vi "SRV_Watchdog State Machine.vi"(7 "Cancelled?":bool, 8 "error in (no error)":errorcluster, 10 "TCP Read semaphore":T1, 11 "SRV IP Address":string) -> (0 "error out":errorcluster)   [LabVIEW 2014]
doc: "Author: Mike Schultz (LogicPD, Inc)"
uses:
  Support/SRV_Command-Data Queue Data Type.ctl
  SRV_Watchdog State Machine Local Data.ctl
  SubVIs/SysConfig/SRV_System Config.ctl
  SRV_Watchdog Config Cluster.ctl
  Motors/Motors Config/SRV_Motor Control Command Config.ctl
  <vilib>/Utility/error.llb/DialogType.ctl
panel:
  out "i":i32
  out "Command History":string[](array[string])
  out "Command":string
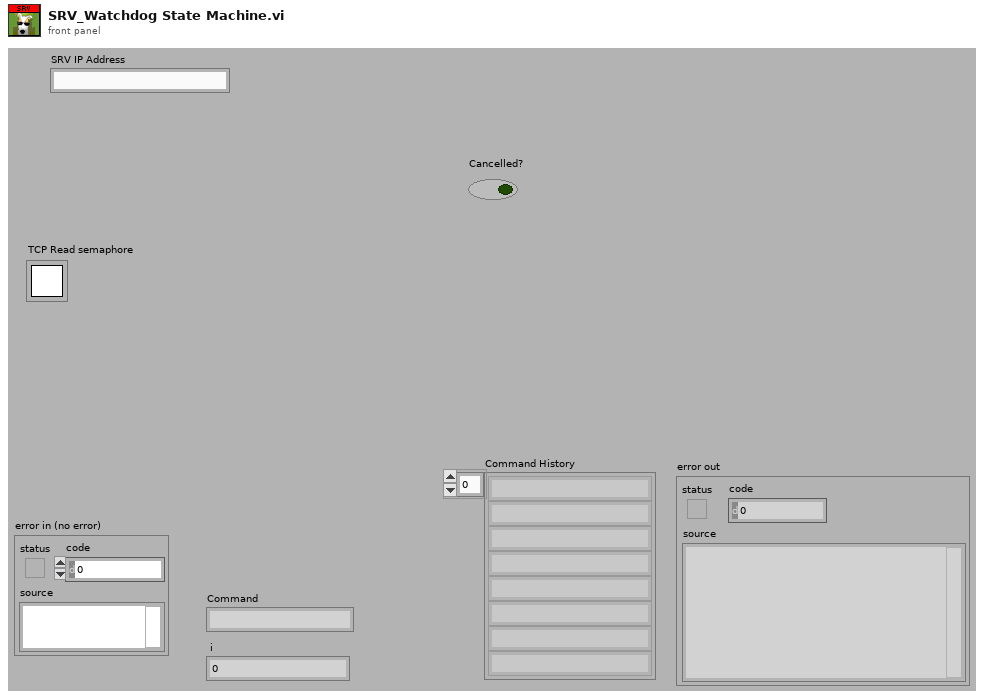
[diagram p1: front panel]
types:
  T1 = typedef "Semaphore RefNum" = refnum<k1>
  T2 = typedef "SRV_Watchdog State Machine Local Data.ctl" = cluster{"SRV IP Address":string, "TCP Read semaphore":T1, "System Config":T3, "WD 1 Last Update":dbl, "WD 2 Last Update":dbl, "SRV":refnum<k5>}
  T3 = typedef "SRV_System Config.ctl" = cluster{"SRV IP Address":string, "Video Stream Rate Period (ms)":u32, "Enable Diagnostic Log":bool, "Watchdog 1 Config":T4, "Watchdog 2 Config":T4, "Sensor Window Filepath":path}
  T4 = typedef "SRV_Watchdog Config Cluster.ctl" = cluster{"Watchdog Name":string, "Watchdog Period (s)":dbl, "Watchdog Command":T5}
  T5 = typedef "SRV_Motor Control Command Config.ctl" = cluster{"I2C Address":u8, "Register":u8, "Value":u8, "Active":bool}
  T6 = typedef "SRV_Command-Data Queue Data Type.ctl" = cluster{"Command":string, "Data":variant}
  T7 = typedef "DialogType.ctl" = u16
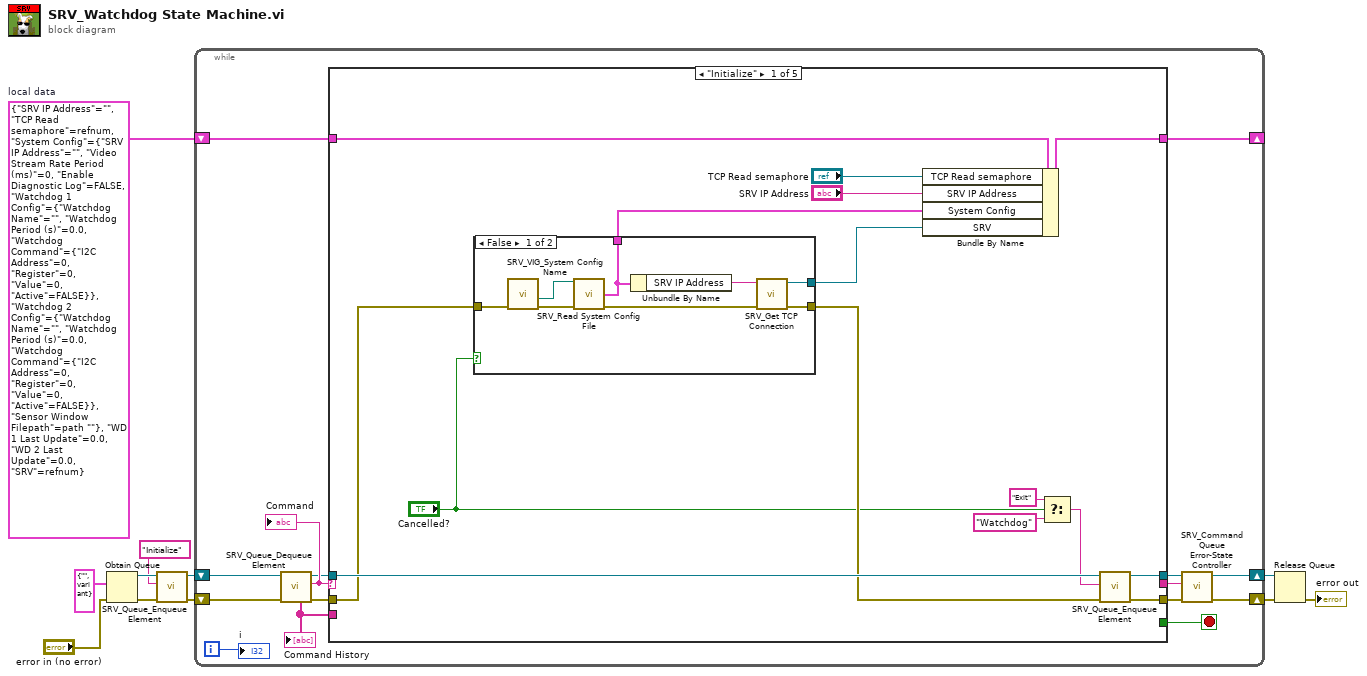
[diagram p0: block diagram]
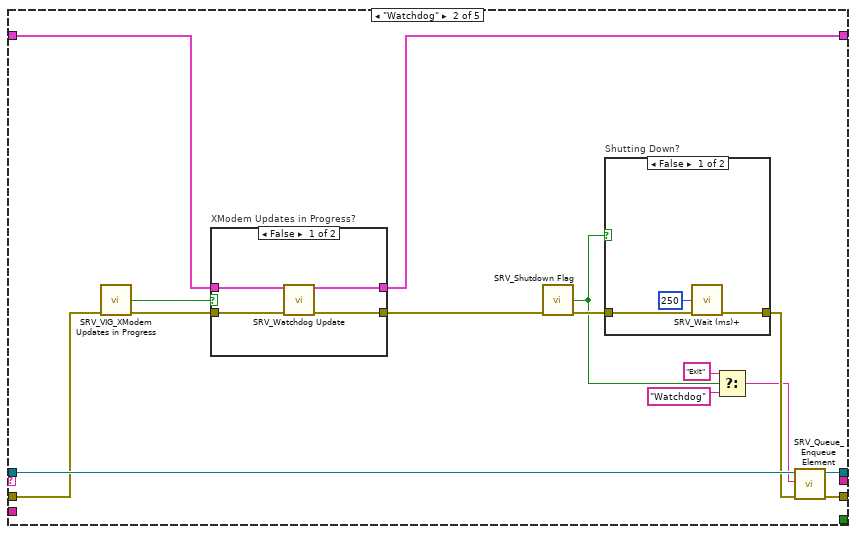
[diagram p3: hidden frame]
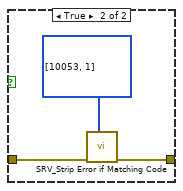
[diagram p5: hidden frame]
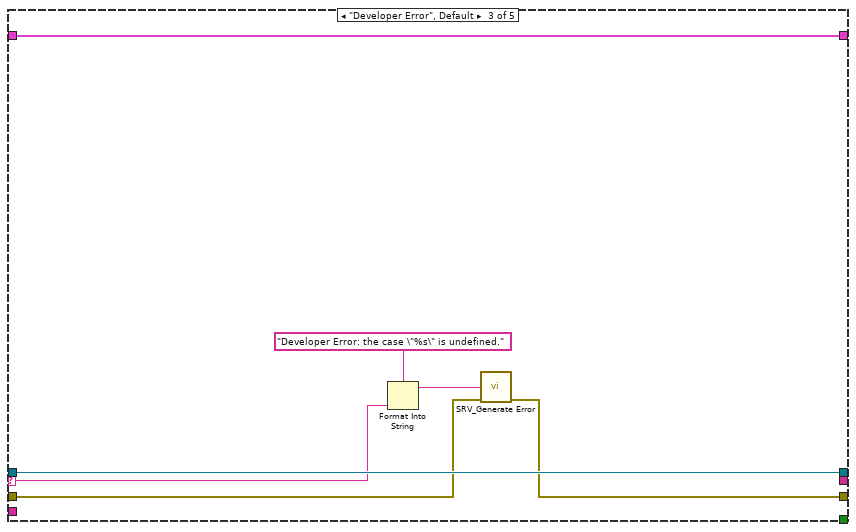
[diagram p6: hidden frame]
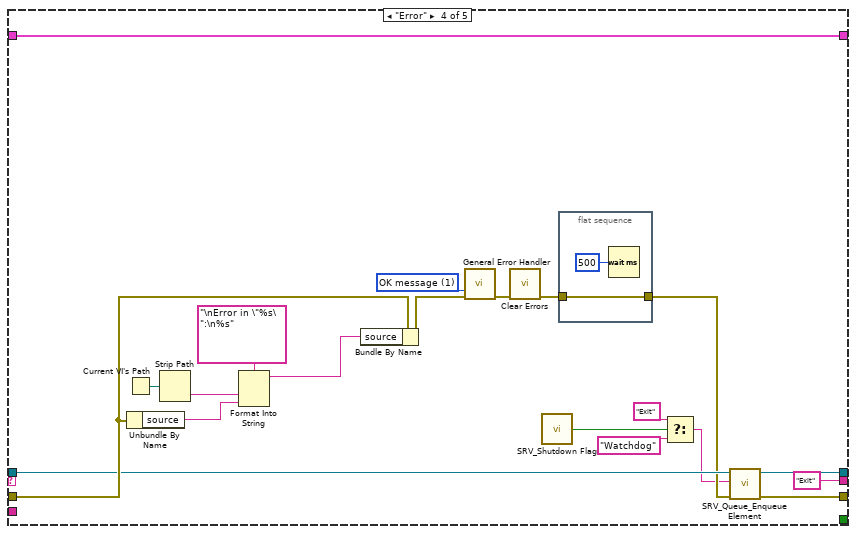
[diagram p7: hidden frame]
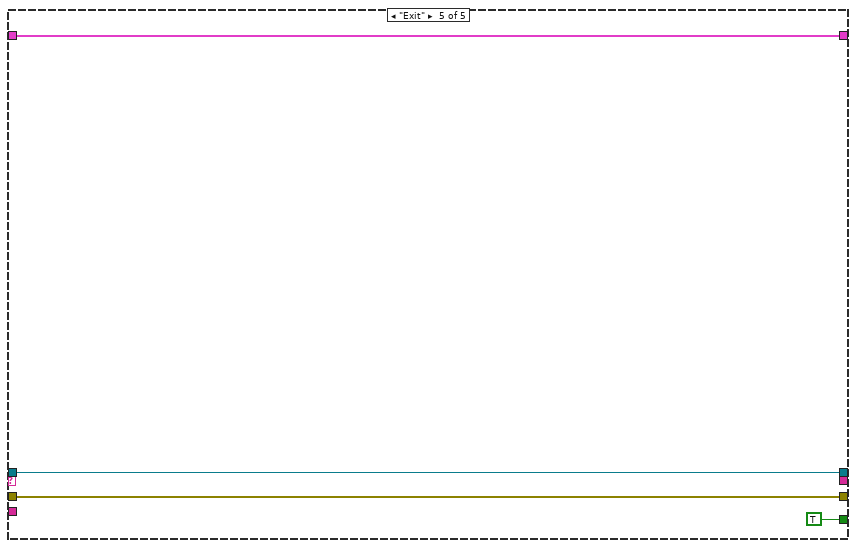
[diagram p8: hidden frame]
diagram:
  w1 = T2 {"SRV IP Address"="", "TCP Read semaphore"=refnum, "System Config"={"SRV IP Address"="", "Video Stream Rate Period (ms)"=0, "Enable Diagnostic Log"=FALSE, "Watchdog 1 Config"={"Watchdog Name"="", "Watchdog Period (s)"=0.0, "Watchdog Command"={"I2C Address"=0, "Register"=0, "Value"=0, "Active"=FALSE}}, "Watchdog 2 Config"={"Watchdog Name"="", "Watchdog Period (s)"=0.0, "Watchdog Command"={"I2C Address"=0, "Register"=0, "Value"=0, "Active"=FALSE}}, "Sensor Window Filepath"=path ""}, "WD 1 Last Update"=0.0, "WD 2 Last Update"=0.0, "SRV"=refnum}  # local data
  n1 = Obtain Queue(element data type=T6 {"Command"="", "Data"=variant} ("Queue Data Type"), error in (no error)="error in (no error)") -> (queue out=w10:refnum<queue>, error out=w8:errorcluster)  [unwired: 3 in, 1 out]
  n2 = call "SRV_Queue_Enqueue Element.vi"("error in (no error)"=w8, "Command"="Initialize", "Command-Data Queue"=w10) -> ("error out"=w7:errorcluster, "Command-Data Queue out"=w9:refnum<queue>)  [unwired: 6 in, 1 out]
  n3 = while {
    shift-right: [w17] -> w4
    shift-left: w7 -> [w24]
    shift-right: [w19] -> w5
    shift-left: w9 -> [w23]
    shift-right: [w14] -> _
    shift-left: w1 -> [w15]
    i -> [w12]
    stop <- w21 stop-if-true
    n4 = call "SRV_Queue_Dequeue Element.vi"("error in (no error)"=w24, "Command-Data Queue"=w23) -> ("error out"=w25:errorcluster, "Command"=w26:string, "Command-Data Queue out"=w22:refnum<queue>, "Command History"=w13:string[])  [unwired: 4 in, 2 out]
    "Command" <- w26
    "Command History" <- w13
    n5 = case shown="\"Initialize\"" w26 {
      selector: w26 -> [_ _ w80 _ _]
      tunnel: w25 -> [w31 w53 w82 w94 w107]
      tunnel: [w41 w64 w83 w93 w107] -> w18
      tunnel: [w40 w65 w84 w91 w110] -> w20
      tunnel: w22 -> [w39 w63 w84 w92 w110]
      tunnel: [_ _ _ _ TRUE] -> w21
      tunnel: [_ _ _ "Exit" ("Error Command") _] -> w16
      tunnel: w15 -> [w38 w56 w78 w103 w108]
      tunnel: [w37 w55 w78 w103 w108] -> w14
      tunnel: w13 -> [_ _ _ _ _]
      frame "Initialize" {
        n6 = case shown="False" "Cancelled?" {
          tunnel: w31 -> [w47 w50]
          tunnel: [w45 w50] -> w30
          tunnel: [w44 _] -> w29
          tunnel: [w42 _] -> w28
          frame False {
            n7 = call "SRV_VIG_System Config Name.vi"("error in (no error)"=w47) -> ("error out"=w49:errorcluster, "SystemConfig Filepath out"=w48:path)  [unwired: 8 in, 1 out]
            n8 = call "SRV_Read System Config File.vi"("System Config File Path"=w48, "error in (no error)"=w49) -> ("System Config"=w44:T3, "error out"=w46:errorcluster)  [unwired: 10 in, 2 out]
            n9 = Unbundle By Name(w44) -> ("SRV IP Address"=w43:string)
            n10 = call "SRV_Get TCP Connection.vi"("error in (no error)"=w46, "IP address"=w43) -> ("error out"=w45:errorcluster, "connection ID"=w42:refnum<k5>)  [unwired: 8 in]
          }
          frame True {
          }
        }
        n11 = Bundle By Name(cluster=w38, "TCP Read semaphore"="TCP Read semaphore", "SRV IP Address"="SRV IP Address", "System Config"=w29, "SRV"=w28) -> (w37:T2)
        n12 = Select(t="Exit" ("Command"), s="Cancelled?", f="Watchdog" ("Command")) -> (s? t:f=w32:string)
        n13 = call "SRV_Queue_Enqueue Element.vi"("error in (no error)"=w30, "Command"=w32, "Command-Data Queue"=w39) -> ("error out"=w41:errorcluster, "Command-Data Queue out"=w40:refnum<queue>)  [unwired: 6 in, 1 out]
      }
      frame "Watchdog" {
        n14 = call "SRV_VIG_XModem Updates in Progress.vi"("error in (no error)"=w53) -> ("XModem Updates in Progress?"=w51:bool, "error out"=w52:errorcluster)  [unwired: 13 in]
        n15 = case "XModem Updates in Progress?" shown="False" w51 {
          tunnel: w56 -> [w69 w70]
          tunnel: [w68 w70] -> w55
          tunnel: [w67 w71] -> w54
          tunnel: w52 -> [w66 w71]
          frame False {
            n16 = call "SRV_Watchdog Update.vi"("Watchdog local data"=w69, "error in (no error)"=w66) -> ("Watchdog local data out"=w68:T2, "error out"=w67:errorcluster)  [unwired: 12 in]
          }
          frame True {
          }
        }
        n17 = call "SRV_Shutdown Flag.vi"("error in (no error)"=w54) -> ("Shutdown Flag out"=w57:bool, "error out"=w62:errorcluster)  [unwired: 13 in]
        n18 = case "Shutting Down?" shown="False" w57 {
          tunnel: w62 -> [w73 w77]
          tunnel: [w72 w76] -> w61
          frame False {
            n19 = call "SRV_Wait (ms)+.vi"("milliseconds to wait"=u32 250, "error in (no error)"=w73) -> ("error out"=w72:errorcluster)  [unwired: 12 in, 1 out]
          }
          frame True {
            n20 = call "SRV_Strip Error if Matching Code.vi"("error in (no error)"=w77, "Strip Codes"=i32[] [10053, 1]) -> ("error out"=w76:errorcluster)  [unwired: 8 in]
          }
        }
        n21 = Select(t="Exit" ("Command"), s=w57, f="Watchdog" ("Command")) -> (s? t:f=w59:string)
        n22 = call "SRV_Queue_Enqueue Element.vi"("error in (no error)"=w61, "Command"=w59, "Command-Data Queue"=w63) -> ("error out"=w64:errorcluster, "Command-Data Queue out"=w65:refnum<queue>)  [unwired: 6 in, 1 out]
      }
      frame "Developer Error", Default {
        n23 = Format Into String(format string="Developer Error: the case \"%s\" is undefined.", w80) -> (resulting string=w81:string)  [unwired: 2 in, 1 out]
        n24 = call "SRV_Generate Error.vi"("Message"=w81, "error in (no error)"=w82) -> ("error out"=w83:errorcluster)  [unwired: 13 in]
      }
      frame "Error" {
        w102 = T7 1 items=["no dialog", "OK message", "continue or stop message", "OK message + warnings", "continue/stop + warnings"] ("type of dialog (OK msg:1)")
        n25 = Current VI's Path() -> (path=w100:path)
        n26 = Unbundle By Name(w94) -> ("source"=w98:string)
        n27 = Strip Path(path=w100) -> (name=w99:string)  [unwired: 1 out]
        n28 = Format Into String(format string="\nError in \"%s\":\n%s", w99, w98) -> (resulting string=w96:string)  [unwired: 2 in, 1 out]
        n29 = Bundle By Name(cluster=w94, "source"=w96) -> (w97:errorcluster)
        n30 = call <vilib>:"General Error Handler.vi"("type of dialog (OK msg:1)"=w102, "error in (no error)"=w97) -> ("error out"=w95:errorcluster)  [unwired: 9 in, 4 out]
        n31 = call <vilib>:"Clear Errors.vi"("error in (no error)"=w95) -> ("error out"=w90:errorcluster)  [unwired: 5 in, 1 out]
        n32 = call "SRV_Shutdown Flag.vi"() -> ("Shutdown Flag out"=w88:bool)  [unwired: 14 in, 1 out]
        n33 = flat-sequence {
          tunnel: w90 -> [w106]
          tunnel: [w106] -> w89
          frame #0 {
            n34 = Wait (ms)(milliseconds to wait=u32 500) -> ()  [unwired: 1 out]
          }
        }
        n35 = Select(t="Exit" ("Command"), s=w88, f="Watchdog" ("Command")) -> (s? t:f=w86:string)
        n36 = call "SRV_Queue_Enqueue Element.vi"("error in (no error)"=w89, "Command"=w86, "Command-Data Queue"=w92) -> ("error out"=w93:errorcluster, "Command-Data Queue out"=w91:refnum<queue>)  [unwired: 6 in, 1 out]
      }
      frame "Exit" {
      }
    }
    n37 = call "SRV_Command Queue Error-State Controller.vi"("error in (no error)"=w18, "Error Command"=w16, "Command-Data Queue"=w20) -> ("error out"=w17:errorcluster, "Command-Data Queue out"=w19:refnum<queue>)  [unwired: 7 in]
    "i" <- w12
  }
  n38 = Release Queue(queue=w5, error in (no error)=w4) -> (error out=→"error out":errorcluster)  [unwired: 1 in, 2 out]
